vi "stage_sim_setup.vi"(11 "serial-numbers":string[](array[string])) -> (3 ".NET Refnum out":refnum<k24>)   [LabVIEW 2024]
uses:
  O:/DSG/Tyler/EIC/DIRC/daq/automated/Thorlabs.MotionControl.DeviceManagerCLI.dll
  Thorlabs.MotionControl.DeviceManagerCLI.dll
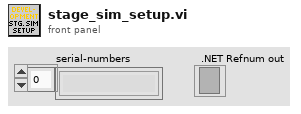
[diagram p1: front panel]
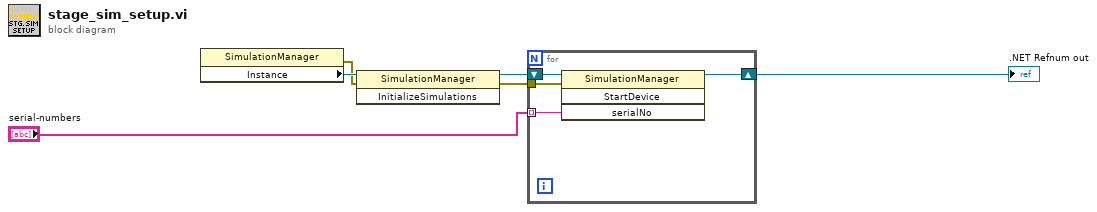
[diagram p0: block diagram]
diagram:
  n1 = property class="SimulationManager"() -> (error out=w2:errorcluster, "Instance"=w4:refnum<k24>)  [unwired: 2 in, 1 out]
  n2 = invoke class="SimulationManager" method="InitializeSimulations"(reference=w4, error in=w2) -> (reference out=w3:refnum<k24>, error out=w1:errorcluster)  [unwired: 1 in, 1 out]
  n3 = for {
    tunnel: w1 -> [w10]
    tunnel: "serial-numbers" -> [w8] mode=indexing
    shift-right: [w7] -> w6
    shift-left: w3 -> [w9]
    n4 = invoke class="SimulationManager" method="StartDevice"(reference=w9, error in=w10, "serialNo"=w8) -> (reference out=w7:refnum<k24>)  [unwired: 1 in, 3 out]
  }
  ".NET Refnum out" <- w6
